vi "XYZThetaGo.vi"(8 "error in (no error)":errorcluster, 10 "XYZTheta In":dbl[](array[numeric]), 11 "Gantry In":refnum<k24>) -> (0 "error out":errorcluster, 2 "XYZTheta Out":dbl[](array[numeric]), 3 "Gantry Out":refnum<k24>)   [LabVIEW 2020, in "Motion.lvclass"]
uses:
  Motion.lvclass
  A3200/A3200.lvclass
  Drivers/Aerotech A3200/Aerotech.lvlib
  C:/Program Files (x86)/Aerotech/A3200/LabVIEW/2010/Bin/Aerotech.A3200.dll
  Program Files (x86)/Aerotech/A3200/LabVIEW/2010/Bin/Aerotech.A3200.dll
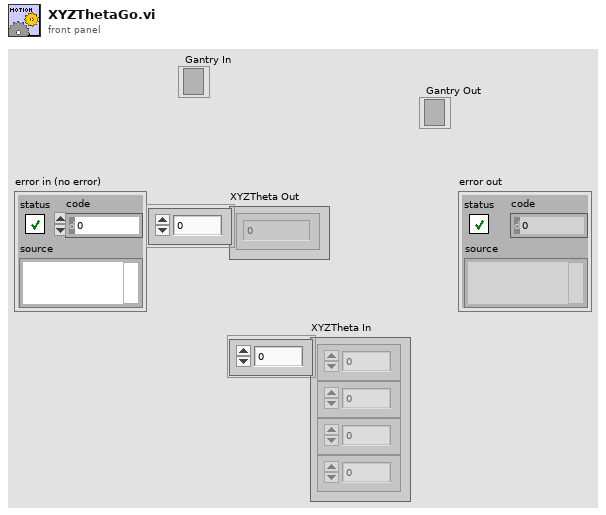
[diagram p1: front panel]
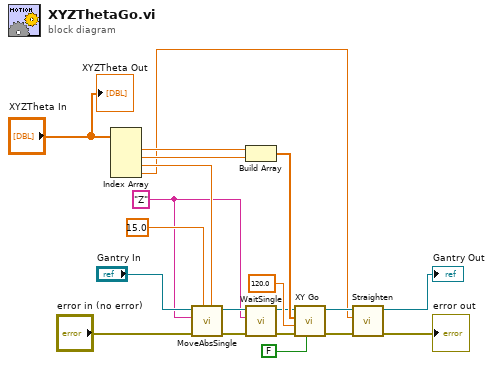
[diagram p0: block diagram]
diagram:
  w7 = "Z" ("axis name")
  n1 = Index Array(array="XYZTheta In") -> (element #1=w16:dbl, element #2=w15:dbl, element #3=w13:dbl, element #4=w2:dbl)  [unwired: 4 in]
  n2 = call "MoveAbsSingle.vi"("position"=w13, "speed"=15.0, "error in (no error)"="error in (no error)", "axis name"=w7, "controller in"="Gantry In") -> ("error out"=w5:errorcluster, "controller out"=w10:refnum<k24>)  [unwired: 5 in]
  n3 = Build Array(w16, w15) -> (w17:dbl[])
  n4 = call "WaitSingle.vi"("error in (no error)"=w5, "axis name"=w7, "controller in"=w10) -> ("error out"=w4:errorcluster, "controller out"=w9:refnum<k24>)  [unwired: 6 in, 1 out]
  n5 = call "XY Go.vi"("return immediately"=FALSE, "error in (no error)"=w4, "Speed"=120.0, "XY In"=w17, "Gantry In"=w9) -> ("error out"=w14:errorcluster, "Gantry Out"=w18:refnum<k24>)  [unwired: 4 in, 1 out]
  n6 = call "Straighten.vi"("error in (no error)"=w14, "Angle (rad)"=w2, "Gantry In"=w18) -> ("error out"=→"error out":errorcluster, "Gantry Out"=→"Gantry Out":refnum<k24>)  [unwired: 7 in]
  "XYZTheta Out" <- "XYZTheta In"
